vi "Vision Research Phantom Series Wait.vi"(11 "Error In (no error)":errorcluster) -> (15 "Error Out":errorcluster)   [LabVIEW 2013, in "VRI.lvlib"]
doc: "NOTE: The wait command is not implemented in the Vision Research Phantom Series camera. This VI will produce an error if used, but has been included as part of the standard driver package in case the command is ever implemented.\n\nThis VI sends a wait command to the instrument to prevent the instrument from executing any futher commands until the current command has finished executing. This may be useful if the instrument needs some time to process a command.\n\nWritten by:\nBLOOMY CONTROLS, INC\nWINDSOR, CT 06095, USA\n860-298-9925\nwww.bloomy.com\nV1.0.0\nMay, 2004"
uses:
  VRI.lvlib
panel:
  # "For instructions on the use of this VI, press Ctrl+H to display the help window and move the mouse over the icon, controls, and indicators"
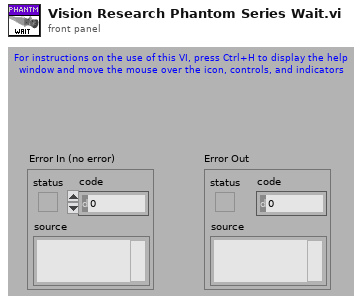
[diagram p1: front panel]
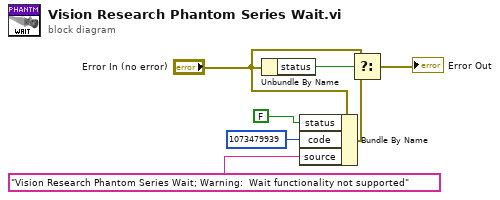
[diagram p0: block diagram]
diagram:
  n1 = Unbundle By Name("Error In (no error)") -> ("status"=w4:bool)
  n2 = Bundle By Name(cluster="Error In (no error)", "status"=FALSE, "code"=1073479939, "source"="Vision Research Phantom Series Wait; Warning:  Wait functionality not supported") -> (w3:errorcluster)
  n3 = Select(t="Error In (no error)", s=w4, f=w3) -> (s? t:f=→"Error Out":errorcluster)
